vi "定点周期设置.vi"(9 "间隔启动":T5 {"启动命令" items=["", "水样测试", "标样核查", "零点核查", "跨度核查", "空白测试", "平行样测试", "加标回收", "空白校准", "标样校准"]}, 10 "定点周期":T2 {"启动命令 24" items=["", "水样测试", "标样核查", "零点核查", "跨度核查", "空白测试", "平行样测试", "加标回收", "空白校准", "标样校准"]; "启动命令 23" items=["", "水样测试", "标样核查", "零点核查", "跨度核查", "空白测试", "平行样测试", "加标回收", "空白校准", "标样校准"]; "启动命令 22" items=["", "水样测试", "标样核查", "零点核查", "跨度核查", "空白测试", "平行样测试", "加标回收", "空白校准", "标样校准"]; "启动命令 21" items=["", "水样测试", "标样核查", "零点核查", "跨度核查", "空白测试", "平行样测试", "加标回收", "空白校准", "标样校准"]; "启动命令 20" items=["", "水样测试", "标样核查", "零点核查", "跨度核查", "空白测试", "平行样测试", "加标回收", "空白校准", "标样校准"]; "启动命令 19" items=["", "水样测试", "标样核查", "零点核查", "跨度核查", "空白测试", "平行样测试", "加标回收", "空白校准", "标样校准"]; "启动命令 18" items=["", "水样测试", "标样核查", "零点核查", "跨度核查", "空白测试", "平行样测试", "加标回收", "空白校准", "标样校准"]; "启动命令 17" items=["", "水样测试", "标样核查", "零点核查", "跨度核查", "空白测试", "平行样测试", "加标回收", "空白校准", "标样校准"]; "启动命令 16" items=["", "水样测试", "标样核查", "零点核查", "跨度核查", "空白测试", "平行样测试", "加标回收", "空白校准", "标样校准"]; "启动命令 15" items=["", "水样测试", "标样核查", "零点核查", "跨度核查", "空白测试", "平行样测试", "加标回收", "空白校准", "标样校准"]; "启动命令 14" items=["", "水样测试", "标样核查", "零点核查", "跨度核查", "空白测试", "平行样测试", "加标回收", "空白校准", "标样校准"]; "启动命令 13" items=["", "水样测试", "标样核查", "零点核查", "跨度核查", "空白测试", "平行样测试", "加标回收", "空白校准", "标样校准"]; "启动命令 12" items=["", "水样测试", "标样核查", "零点核查", "跨度核查", "空白测试", "平行样测试", "加标回收", "空白校准", "标样校准"]; "启动命令 11" items=["", "水样测试", "标样核查", "零点核查", "跨度核查", "空白测试", "平行样测试", "加标回收", "空白校准", "标样校准"]; "启动命令 10" items=["", "水样测试", "标样核查", "零点核查", "跨度核查", "空白测试", "平行样测试", "加标回收", "空白校准", "标样校准"]; "启动命令 9" items=["", "水样测试", "标样核查", "零点核查", "跨度核查", "空白测试", "平行样测试", "加标回收", "空白校准", "标样校准"]; "启动命令 8" items=["", "水样测试", "标样核查", "零点核查", "跨度核查", "空白测试", "平行样测试", "加标回收", "空白校准", "标样校准"]; "启动命令 7" items=["", "水样测试", "标样核查", "零点核查", "跨度核查", "空白测试", "平行样测试", "加标回收", "空白校准", "标样校准"]; "启动命令 6" items=["", "水样测试", "标样核查", "零点核查", "跨度核查", "空白测试", "平行样测试", "加标回收", "空白校准", "标样校准"]; "启动命令 5" items=["", "水样测试", "标样核查", "零点核查", "跨度核查", "空白测试", "平行样测试", "加标回收", "空白校准", "标样校准"]; "启动命令 4" items=["", "水样测试", "标样核查", "零点核查", "跨度核查", "空白测试", "平行样测试", "加标回收", "空白校准", "标样校准"]; "启动命令 3" items=["", "水样测试", "标样核查", "零点核查", "跨度核查", "空白测试", "平行样测试", "加标回收", "空白校准", "标样校准"]; "启动命令 2" items=["", "水样测试", "标样核查", "零点核查", "跨度核查", "空白测试", "平行样测试", "加标回收", "空白校准", "标样校准"]; "启动命令" items=["", "水样测试", "标样核查", "零点核查", "跨度核查", "空白测试", "平行样测试", "加标回收", "空白校准", "标样校准"]}, 11 "周期模式":T1) -> (2 "保存输出":bool, 3 "周期设置输出":T4 {"定点周期"."启动命令 24" items=["", "水样测试", "标样核查", "零点核查", "跨度核查", "空白测试", "平行样测试", "加标回收", "空白校准", "标样校准"]; "定点周期"."启动命令 23" items=["", "水样测试", "标样核查", "零点核查", "跨度核查", "空白测试", "平行样测试", "加标回收", "空白校准", "标样校准"]; "定点周期"."启动命令 22" items=["", "水样测试", "标样核查", "零点核查", "跨度核查", "空白测试", "平行样测试", "加标回收", "空白校准", "标样校准"]; "定点周期"."启动命令 21" items=["", "水样测试", "标样核查", "零点核查", "跨度核查", "空白测试", "平行样测试", "加标回收", "空白校准", "标样校准"]; "定点周期"."启动命令 20" items=["", "水样测试", "标样核查", "零点核查", "跨度核查", "空白测试", "平行样测试", "加标回收", "空白校准", "标样校准"]; "定点周期"."启动命令 19" items=["", "水样测试", "标样核查", "零点核查", "跨度核查", "空白测试", "平行样测试", "加标回收", "空白校准", "标样校准"]; "定点周期"."启动命令 18" items=["", "水样测试", "标样核查", "零点核查", "跨度核查", "空白测试", "平行样测试", "加标回收", "空白校准", "标样校准"]; "定点周期"."启动命令 17" items=["", "水样测试", "标样核查", "零点核查", "跨度核查", "空白测试", "平行样测试", "加标回收", "空白校准", "标样校准"]; "定点周期"."启动命令 16" items=["", "水样测试", "标样核查", "零点核查", "跨度核查", "空白测试", "平行样测试", "加标回收", "空白校准", "标样校准"]; "定点周期"."启动命令 15" items=["", "水样测试", "标样核查", "零点核查", "跨度核查", "空白测试", "平行样测试", "加标回收", "空白校准", "标样校准"]; "定点周期"."启动命令 14" items=["", "水样测试", "标样核查", "零点核查", "跨度核查", "空白测试", "平行样测试", "加标回收", "空白校准", "标样校准"]; "定点周期"."启动命令 13" items=["", "水样测试", "标样核查", "零点核查", "跨度核查", "空白测试", "平行样测试", "加标回收", "空白校准", "标样校准"]; "定点周期"."启动命令 12" items=["", "水样测试", "标样核查", "零点核查", "跨度核查", "空白测试", "平行样测试", "加标回收", "空白校准", "标样校准"]; "定点周期"."启动命令 11" items=["", "水样测试", "标样核查", "零点核查", "跨度核查", "空白测试", "平行样测试", "加标回收", "空白校准", "标样校准"]; "定点周期"."启动命令 10" items=["", "水样测试", "标样核查", "零点核查", "跨度核查", "空白测试", "平行样测试", "加标回收", "空白校准", "标样校准"]; "定点周期"."启动命令 9" items=["", "水样测试", "标样核查", "零点核查", "跨度核查", "空白测试", "平行样测试", "加标回收", "空白校准", "标样校准"]; "定点周期"."启动命令 8" items=["", "水样测试", "标样核查", "零点核查", "跨度核查", "空白测试", "平行样测试", "加标回收", "空白校准", "标样校准"]; "定点周期"."启动命令 7" items=["", "水样测试", "标样核查", "零点核查", "跨度核查", "空白测试", "平行样测试", "加标回收", "空白校准", "标样校准"]; "定点周期"."启动命令 6" items=["", "水样测试", "标样核查", "零点核查", "跨度核查", "空白测试", "平行样测试", "加标回收", "空白校准", "标样校准"]; "定点周期"."启动命令 5" items=["", "水样测试", "标样核查", "零点核查", "跨度核查", "空白测试", "平行样测试", "加标回收", "空白校准", "标样校准"]; "定点周期"."启动命令 4" items=["", "水样测试", "标样核查", "零点核查", "跨度核查", "空白测试", "平行样测试", "加标回收", "空白校准", "标样校准"]; "定点周期"."启动命令 3" items=["", "水样测试", "标样核查", "零点核查", "跨度核查", "空白测试", "平行样测试", "加标回收", "空白校准", "标样校准"]; "定点周期"."启动命令 2" items=["", "水样测试", "标样核查", "零点核查", "跨度核查", "空白测试", "平行样测试", "加标回收", "空白校准", "标样校准"]; "定点周期"."启动命令" items=["", "水样测试", "标样核查", "零点核查", "跨度核查", "空白测试", "平行样测试", "加标回收", "空白校准", "标样校准"]; "间隔设置"."启动命令" items=["", "水样测试", "标样核查", "零点核查", "跨度核查", "空白测试", "平行样测试", "加标回收", "空白校准", "标样校准"]})   [LabVIEW 2016, in "定时设置.xctl"]
panel:
  in  "保存":bool
  in  "退出":bool
  in  "清空":bool
  out "周期模式选择卡":enum32{"选项卡 1", "选项卡 2"}(tab)
  # "分钟"
  # "次"
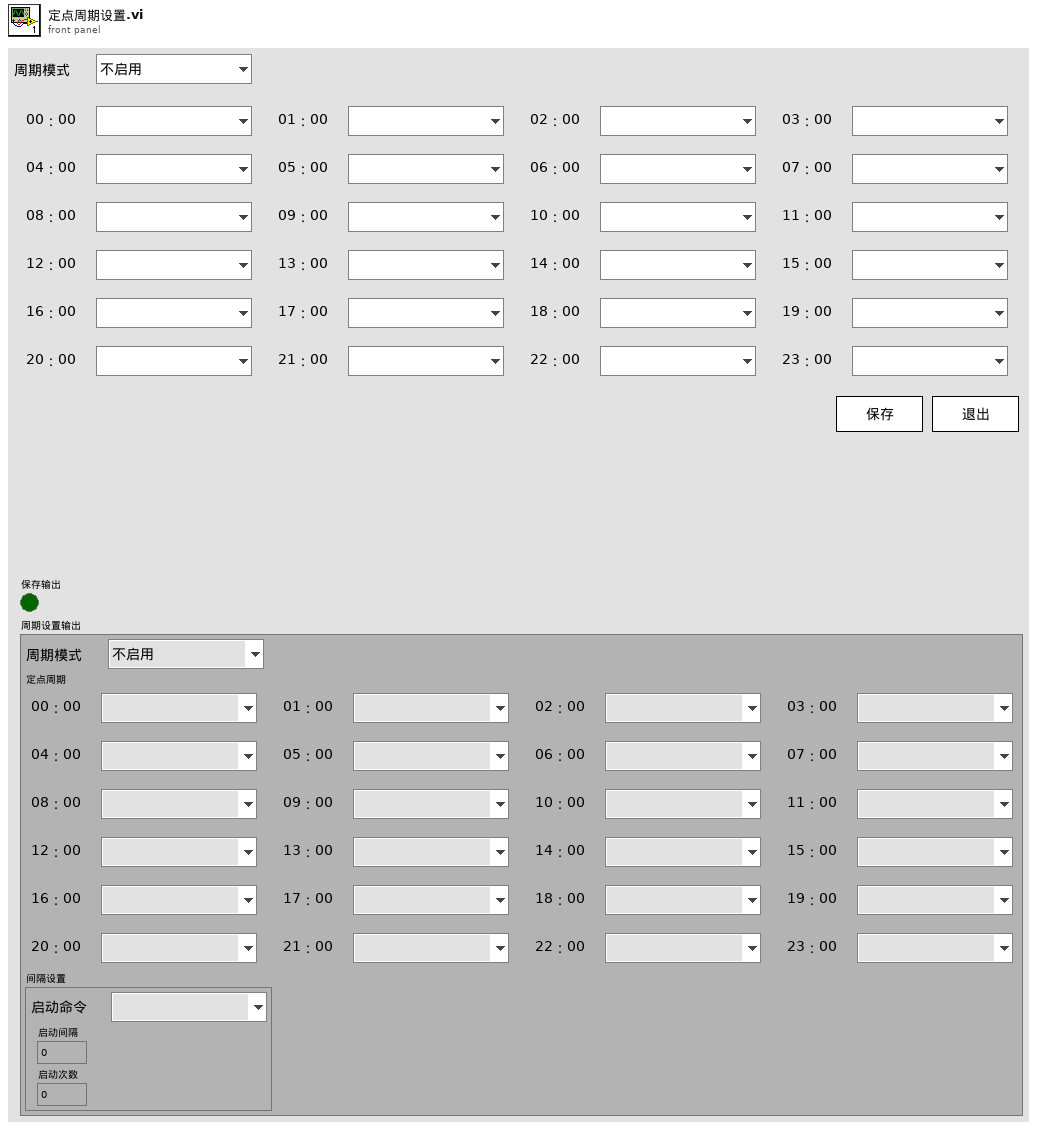
[diagram p1: front panel]
types:
  T1 = typedef "定时设置.xctl/周期模式设置.ctl" = enum16{"不启用", "定点模式", "间隔模式"}
  T2 = typedef "定时设置.xctl/定点周期设置.ctl" = cluster{"启动命令":T3, "启动命令 2":T3, "启动命令 3":T3, "启动命令 4":T3, "启动命令 5":T3, "启动命令 6":T3, "启动命令 7":T3, "启动命令 8":T3, "启动命令 9":T3, "启动命令 10":T3, "启动命令 11":T3, "启动命令 12":T3, "启动命令 13":T3, "启动命令 14":T3, "启动命令 15":T3, "启动命令 16":T3, "启动命令 17":T3, "启动命令 18":T3, "启动命令 19":T3, "启动命令 20":T3, "启动命令 21":T3, "启动命令 22":T3, "启动命令 23":T3, "启动命令 24":T3}
  T3 = typedef "定时设置.xctl/启动命令选择.ctl" = u16
  T4 = cluster{"周期模式":T1, "定点周期":T2, "间隔设置":cluster{"启动命令":T3, "启动间隔":dbl, "启动次数":i32}}
  T5 = typedef "定时设置.xctl/间隔启动设置.ctl" = cluster{"启动命令":T3, "启动间隔":dbl, "启动次数":i32}
  T6 = typedef "周期设置.lvlib/周期模式设置.ctl" = enum16{"不启用", "定点模式", "间隔模式"}
  T7 = cluster{"周期模式":T1, "定点周期":T2, cluster{"启动命令":T3, "启动间隔":dbl, "启动次数":i32}}
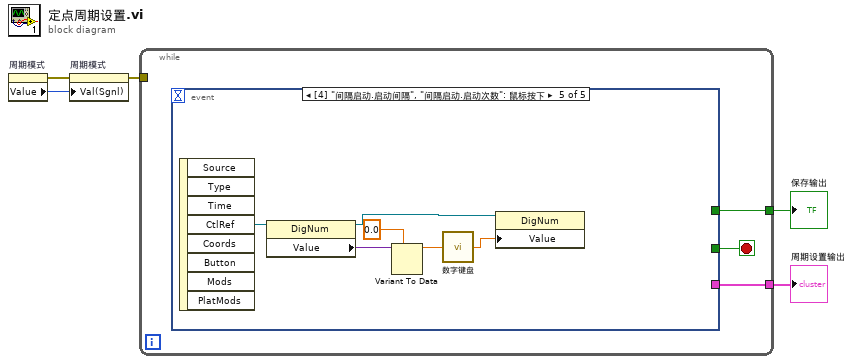
[diagram p0: block diagram]
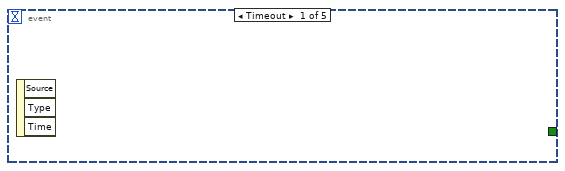
[diagram p2: hidden frame]
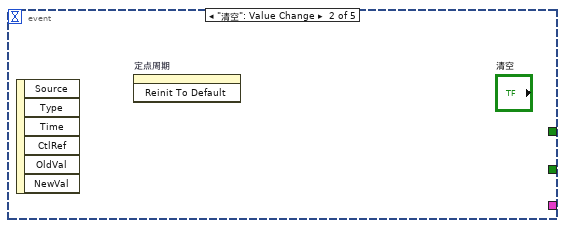
[diagram p3: hidden frame]
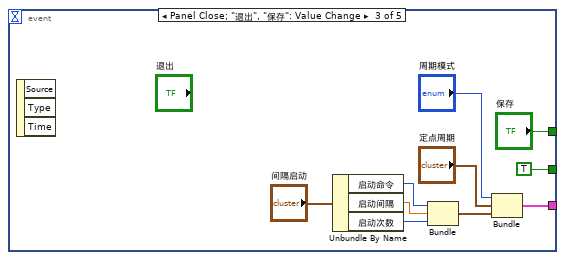
[diagram p4: hidden frame]
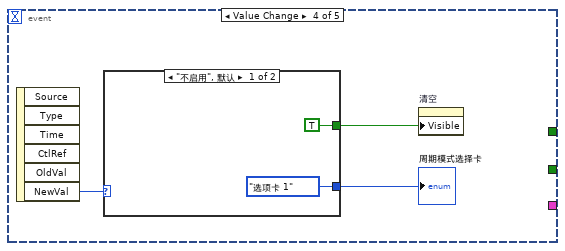
[diagram p5: hidden frame]
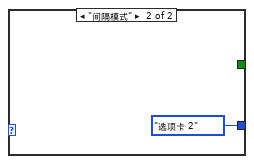
[diagram p6: hidden frame]
diagram:
  n1 = property on="周期模式" class="Enum (严格)"() -> (error out=w4:errorcluster, "Value"=w5:T6)  [unwired: 2 in, 1 out]
  n2 = property on="周期模式" class="Enum (严格)"(error in=w4, "Val(Sgnl)"=w5) -> (error out=w3:errorcluster)  [unwired: 1 in, 1 out]
  n3 = while {
    tunnel: [w7] -> w2
    tunnel: w3 -> [_]
    tunnel: [w6] -> w1
    stop <- w8 stop-if-true
    n4 = event shown="[4] \"间隔启动.启动间隔\", \"间隔启动.启动次数\": 鼠标按下" {
      selector: _ -> [_ _ _ _ _]
      dyn-events: _ -> [_ _ _ _ _]
      timeout: _ -> [_ _ _ _ _]
      tunnel: [_ _ TRUE _ _] -> w8
      tunnel: [_ _ w17 _ _] -> w7
      tunnel: [_ _ "保存" _ _] -> w6
      event Timeout {
        n5 = event-data() -> ()  [unwired: 1 in, 3 out]
      }
      event "清空": Value Change {
        n6 = event-data() -> ()  [unwired: 1 in, 6 out]
        n7 = invoke on="定点周期" class="Clust (严格)" method="Reinit To Default"() -> ()  [unwired: 3 in, 3 out]
      }
      event Panel Close; "退出", "保存": Value Change {
        n8 = event-data() -> ()  [unwired: 1 in, 3 out]
        n9 = Unbundle By Name("间隔启动") -> ("启动命令"=w14:T3, "启动间隔"=w13:dbl, "启动次数"=w12:i32)
        n10 = Bundle("启动命令"=w14, "启动间隔"=w13, "启动次数"=w12) -> (w11:cluster{"启动命令":T3, "启动间隔":dbl, "启动次数":i32})  [unwired: 1 in]
        n11 = Bundle("周期模式"="周期模式", "定点周期"="定点周期", w11) -> (w17:T7)  [unwired: 1 in]
      }
      event Value Change {
        n12 = event-data() -> ("NewVal"=w20:T1)  [unwired: 1 in, 5 out]
        n13 = case shown="\"不启用\", 默认" w20 {
          tunnel: [TRUE ("可见") _] -> w21
          tunnel: [enum32{"选项卡 1", "选项卡 2"}."选项卡 1" ("周期模式选择卡") enum32{"选项卡 1", "选项卡 2"}."选项卡 2" ("周期模式选择卡")] -> w19
          frame "不启用", Default {
          }
          frame "间隔模式" {
          }
        }
        "周期模式选择卡" <- w19
        n14 = property on="清空" class="Bool"("Visible"=w21) -> ()  [unwired: 2 in, 2 out]
      }
      event Mouse Down {
        n15 = event-data() -> ("CtlRef"=w30:refnum<vi>)  [unwired: 1 in, 7 out]
        n16 = property class="DigNum"(reference=w30) -> (reference out=w29:refnum<vi>, "Value"=w28:variant)  [unwired: 1 in, 1 out]
        n17 = Variant To Data(type=0.0, Variant=w28) -> (data=w26:dbl)  [unwired: 1 in, 1 out]
        n18 = call "数字键盘.vi"("OldNumber"=w26) -> ("NewNumber"=w25:sgl)
        n19 = property class="DigNum"(reference=w29, "Value"=w25) -> ()  [unwired: 1 in, 2 out]
      }
    }
  }
  "周期设置输出" <- w2
  "保存输出" <- w1
